vi "PH_SHS_Analysis.evt call Read Cali Data.vi"(0 "i ref in":refnum<vi>, 1 "Instance":string, 2 "Cali Data File":path, 5 "error in (no error)":errorcluster) -> (14 "i ref out":refnum<vi>, 19 "error out":errorcluster)   [LabVIEW 2014, in "PH_SHS_Analysis.lvlib"]
doc: "This VI calls the event case \"ReadCaliData\" by a simple call."
uses:
  PH_SHS_Analysis.lvlib
  CS_Core/CSSystem/CoreLib/CoreLib.string 2 byte array.vi
  CS_Core/CSSystem/CoreLib/CoreLib.lvlib
  CS_Core/BaseProcess/BaseProcess.lvlib
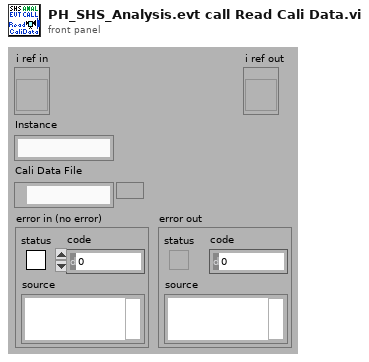
[diagram p1: front panel]
types:
  T1 = typedef "CoreDefs.rawDataType.ctl" = i8[]
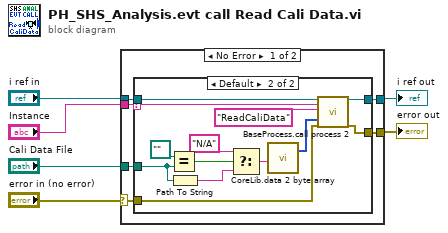
[diagram p0: block diagram]
diagram:
  n1 = case shown="No Error" "error in (no error)" {
    selector: "error in (no error)" -> [w9 w28]
    tunnel: [w12 w29] -> w2
    tunnel: [w11 w28] -> w1
    tunnel: "i ref in" -> [w10 w29]
    tunnel: "Instance" -> [w8 _]
    tunnel: "Cali Data File" -> [w7 _]
    frame No Error {
      n2 = case shown="Default" w8 {
        selector: w8 -> [_ w21]
        tunnel: [w14 w26] -> w12
        tunnel: [w13 w25] -> w11
        tunnel: w10 -> [w14 w24]
        tunnel: w9 -> [w13 w22]
        tunnel: w7 -> [_ w19]
        frame "N/A" {
        }
        frame Default {
          n3 = Equal?(x=path "" ("Cali Data File"), y=w19) -> (x = y?=w18:bool)
          n4 = Path To String(path=w19) -> (string=w17:string)
          n5 = Select(t="N/A", s=w18, f=w17) -> (s? t:f=w16:string)
          n6 = call-poly "CoreLib.data 2 byte array.vi"("string"=w16) -> ("byteArray out"=w23:T1)  [unwired: 18 in]
          n7 = call "BaseProcess.call process 2.vi"("i ref in"=w24, "Object"=w21, "Selector"="ReadCaliData", "Data"=w23, "error in (no error)"=w22) -> ("i ref out"=w26:refnum<vi>, "error out"=w25:errorcluster)  [unwired: 13 in]
        }
      }
    }
    frame Error {
    }
  }
  "i ref out" <- w2
  "error out" <- w1
